vi "Draw Circle.vi"(4 "Drawing Mode":u32(ring)=1 items=["Frame", "Fill"], 6 "Radius":i32, 7 "Object Color":u32, 8 "error in (no error)":errorcluster, 9 "Y":i32, 10 "X":i32, 11 "Refnum in":T1) -> (0 "error out":errorcluster, 3 "Refnum out":T1)   [LabVIEW 2016]
uses:
  <vilib>/vision/Image Controls.llb/IMAQ Image.ctl
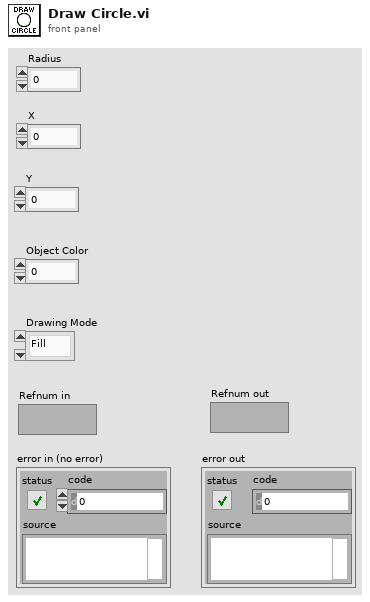
[diagram p1: front panel]
types:
  T1 = typedef "IMAQ Image.ctl" = refnum<image>
  T2 = cluster{"X Resolution":i32, "Y Resolution":i32, "X Resolution":i32, "Y Resolution":i32}
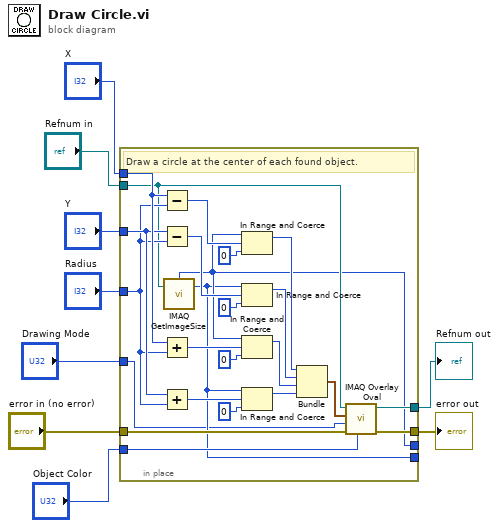
[diagram p0: block diagram]
diagram:
  n1 = in-place {
    in-place-border: "Refnum in" -> [w13]
    in-place-border: [w33] -> w6
    in-place-border: [w32] -> w7
    in-place-border: [w12] -> _
    in-place-border: [w11] -> _
    in-place-border: "X" -> [w22]
    in-place-border: "Y" -> [w21]
    in-place-border: "Radius" -> [w16]
    in-place-border: "error in (no error)" -> [w15]
    in-place-border: "Object Color" -> [w14]
    in-place-border: "Drawing Mode" -> [w10]
    # "Draw a circle at the center of each found object."
    n2 = Subtract(x=w22, y=w16) -> (x-y=w20:i32)
    n3 = Subtract(x=w21, y=w16) -> (x-y=w18:i32)
    n4 = Add(x=w22, y=w16) -> (x+y=w19:i32)
    n5 = Add(x=w21, y=w16) -> (x+y=w17:i32)
    n6 = call "IMAQ GetImageSize"("Image"=w13) -> ("Y Resolution"=w11:i32, "X Resolution"=w12:i32)  [unwired: 3 in, 1 out]
    n7 = In Range and Coerce(upper limit=w12, x=w20, lower limit=0) -> (coerced(x)=w30:i32)  [unwired: 1 out]
    n8 = In Range and Coerce(upper limit=w11, x=w18, lower limit=0) -> (coerced(x)=w28:i32)  [unwired: 1 out]
    n9 = In Range and Coerce(upper limit=w12, x=w19, lower limit=0) -> (coerced(x)=w26:i32)  [unwired: 1 out]
    n10 = In Range and Coerce(upper limit=w11, x=w17, lower limit=0) -> (coerced(x)=w24:i32)  [unwired: 1 out]
    n11 = Bundle("X Resolution"=w30, "Y Resolution"=w28, "X Resolution"=w26, "Y Resolution"=w24) -> (w23:T2)  [unwired: 1 in]
    n12 = call "IMAQ Overlay Oval"("Color"=w14, "error in (no error)"=w15, "Drawing Mode (Frame)"=w10, "Bounding Rectangle"=w23, "Image"=w13) -> ("error out"=w32:errorcluster, "Image Out"=w33:T1)  [unwired: 5 in]
  }
  "error out" <- w7
  "Refnum out" <- w6
